vi "SERIAL_RawDataGlobal.vi"(10 "Set":bool=TRUE, 11 "RawData":T1) -> (3 "RawData 2":T1)   [LabVIEW 2014, in "navX-MXP IMU.lvlib"]
uses:
  navX-MXP IMU.lvlib
  TypeDefs/navX Raw Data.ctl
  COMMON/TypeDefs/Data TypeDefs/navX Vector Data.ctl
  <vilib>/Rock Robotics/SystemInterfaces/Utilities/FPGA_UtilitiesRead LocalTime.vi
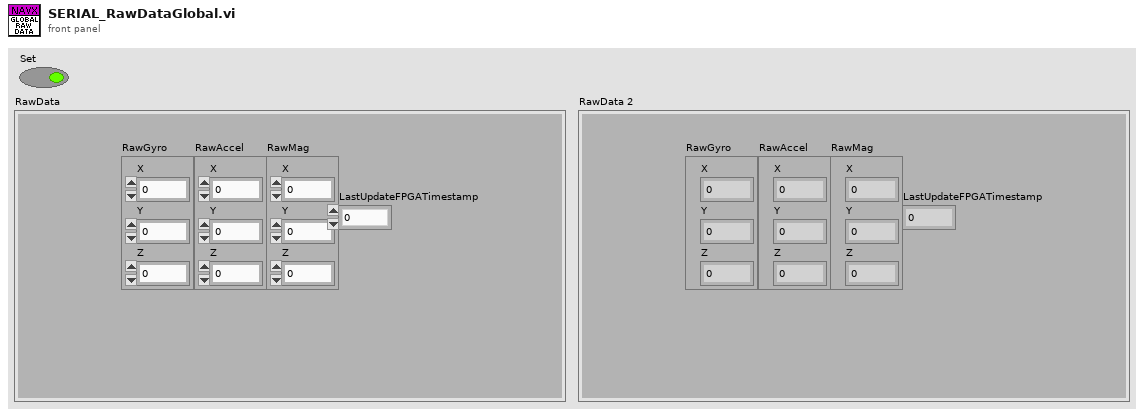
[diagram p1: front panel]
types:
  T1 = typedef "navX-MXP IMU.lvlib/navX Raw Data.ctl" = cluster{"RawAccel":T2, "RawGyro":T2, "RawMag":T2, "LastUpdateFPGATimestamp":dbl}
  T2 = typedef "navX-MXP IMU.lvlib/navX Vector Data.ctl" = cluster{"X":dbl, "Y":dbl, "Z":dbl}
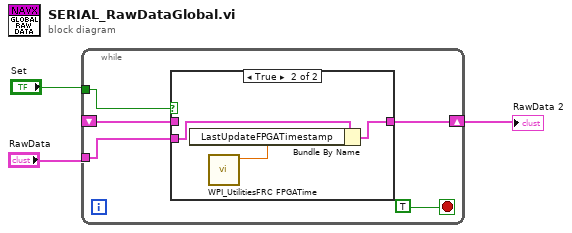
[diagram p0: block diagram]
diagram:
  n1 = while {
    shift-right: [w5] -> w1
    shift-left: _ -> [w4]
    tunnel: "RawData" -> [w6]
    tunnel: "Set" -> [w7]
    stop <- TRUE stop-if-true
    n2 = case shown="True" w7 {
      tunnel: w6 -> [_ w12]
      tunnel: [w9 w10] -> w5
      tunnel: w4 -> [w9 _]
      frame False {
      }
      frame True {
        n3 = call <vilib>:"WPI_UtilitiesFRC FPGATime.vi"() -> ("FPGA Time"=w11:dbl)  [unwired: 10 in, 1 out]
        n4 = Bundle By Name(cluster=w12, "LastUpdateFPGATimestamp"=w11) -> (w10:T1)
      }
    }
  }
  "RawData 2" <- w1
